vi "Hard Link To Source.vi"(8 "Error In":errorcluster, 11 "Configuration in":T1) -> (0 "Error Out":errorcluster, 2 "Files Added To Source":path[](array[path]), 3 "Configuration out":T1)   [LabVIEW 2011, in "LVH-Build-Tools.lvlib"]
doc: "Scan through all components and create hardlinks in source for any files that exist in install but not source."
uses:
  <vilib>/LabVIEW Hacker/Build Tools/LVH-Build-Tools.lvlib
  Type Defs/Configuration.ctl
  Type Defs/Install Configuration.ctl
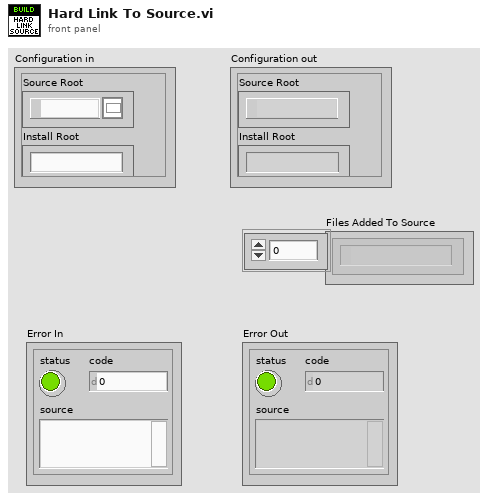
[diagram p1: front panel]
types:
  T1 = typedef "LVH-Build-Tools.lvlib/Configuration.ctl" = cluster{"Source Root":path, "Install Root":string, "Components":string[], "Ignore":string[], "Config Files":path[], "LV Directories":path[], "Install Paths":T2}
  T2 = typedef "LVH-Build-Tools.lvlib/Install Configuration.ctl" = cluster{"LabVIEW Directory":path, "Project Source Config":path}
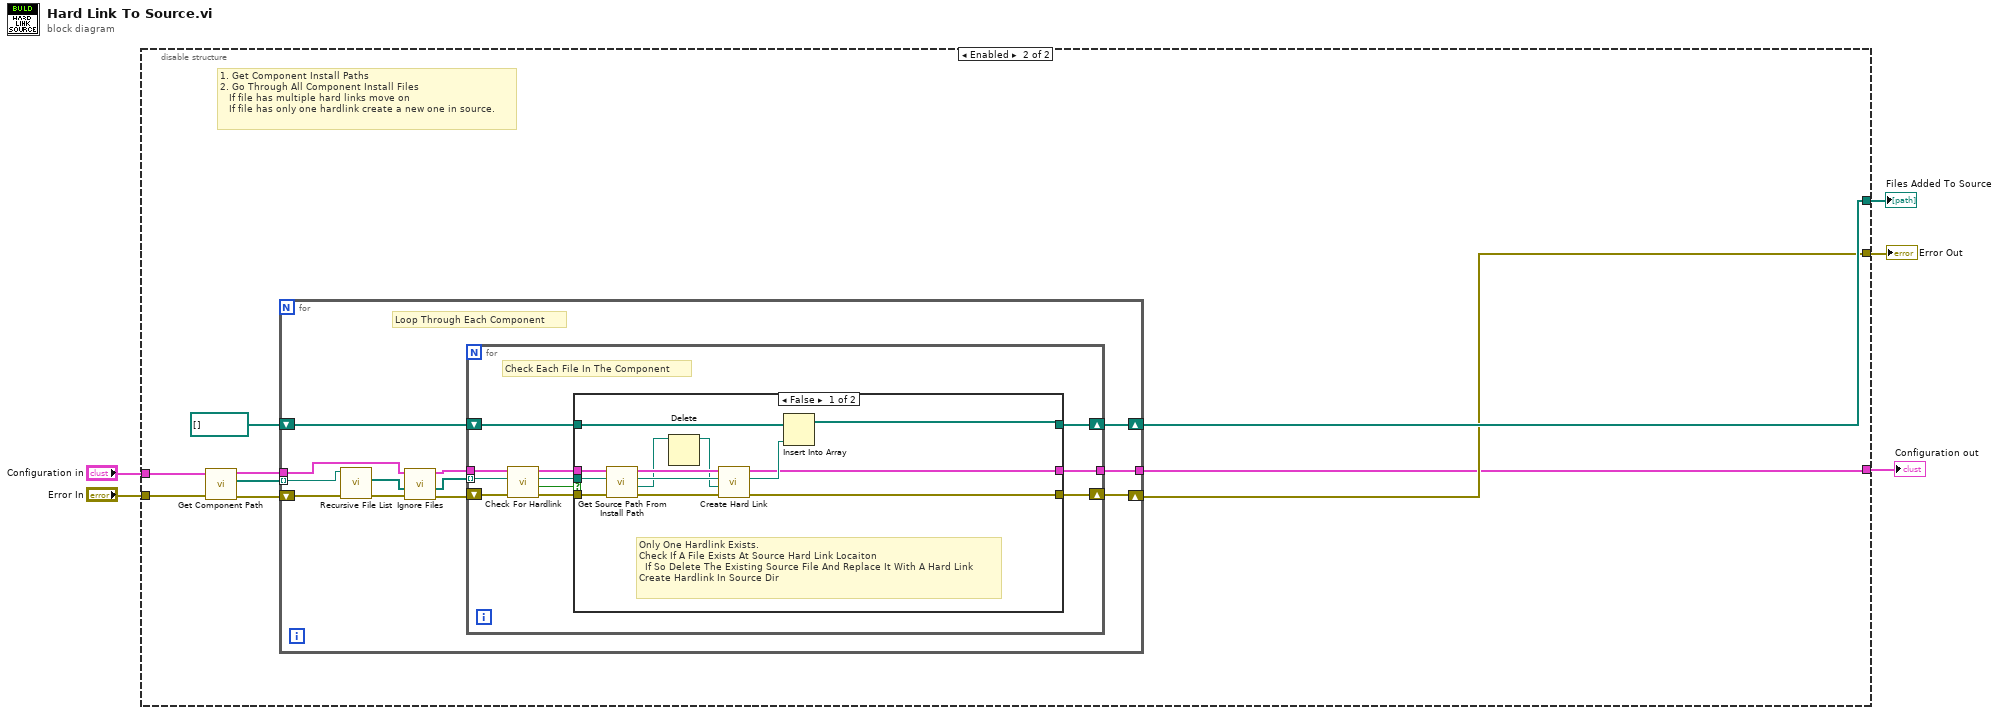
[diagram p0: block diagram]
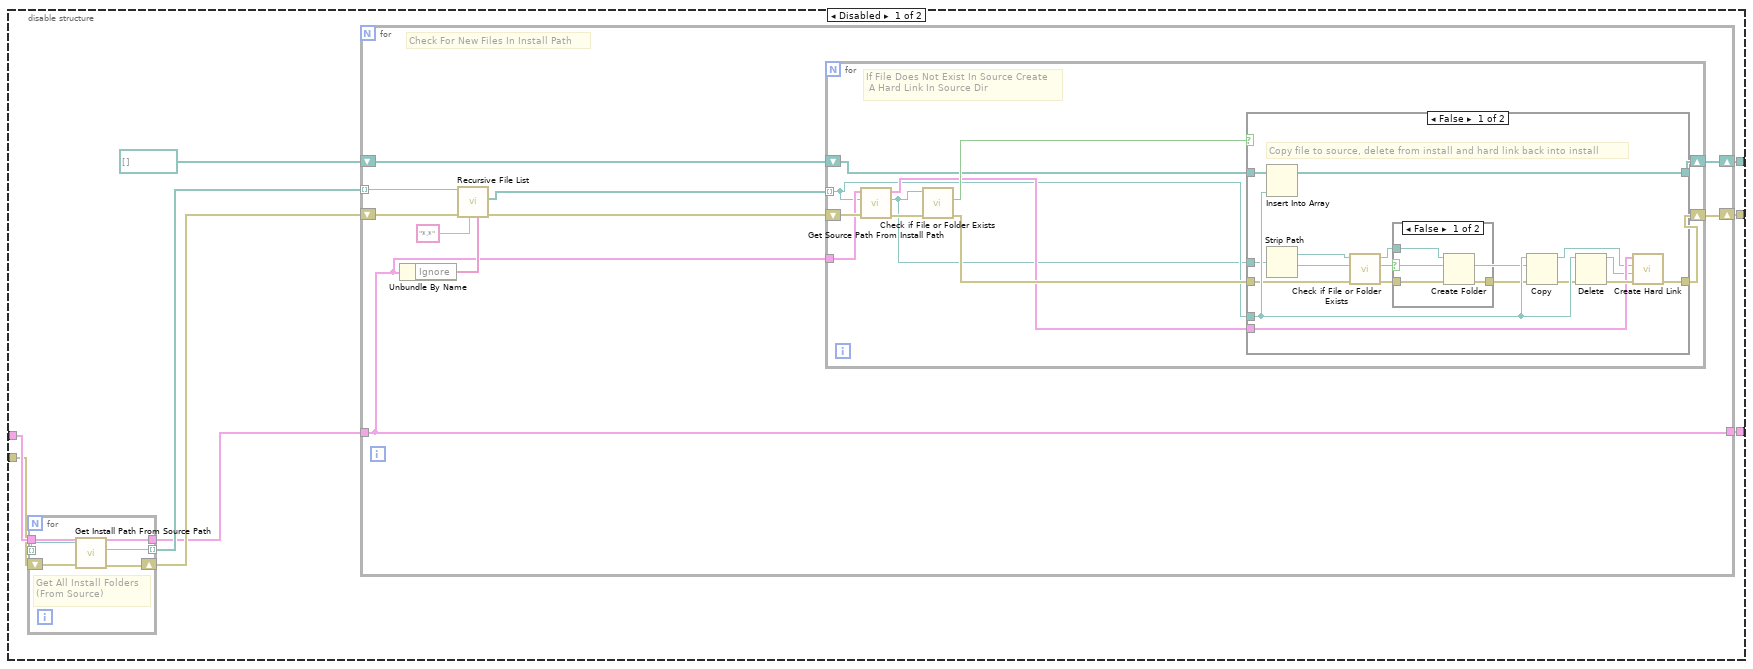
[diagram p2: hidden frame]
diagram:
  n1 = disable-structure shown="Enabled" {
    disable-tunnel: "Configuration in" -> [w11 w73]
    disable-tunnel: "Error In" -> [w10 w72]
    disable-tunnel: [w9 w65] -> w3
    disable-tunnel: [w8 w66] -> w2
    disable-tunnel: [w7 w67] -> w1
    frame Disabled {
      n2 = for {
        tunnel: w11 -> [w20]
        tunnel: [w19] -> w12
        tunnel: [w17] -> w14 mode=indexing
        shift-right: [w18] -> w13
        shift-left: w10 -> [w21]
        tunnel: [w16] -> w15 mode=indexing
        # "Get All Install Folders \n(From Source)"
        n3 = call "Get Install Path From Source Path.vi"("Error In"=w21, "Source File Path"=w17, "Configuration"=w20) -> ("Error Out"=w18:errorcluster, "Install File Path"=w16:path, "Configuration"=w19:T1)  [unwired: 5 in, 1 out]
      }
      n4 = for {
        tunnel: w15 -> [w31] mode=indexing
        shift-right: [w25] -> w8
        shift-left: w13 -> [w30]
        tunnel: w12 -> [w22]
        tunnel: [w22] -> w9
        shift-right: [w23] -> w7
        shift-left: path[] [] -> [w24]
        # "Check For New Files In Install Path"
        n5 = Unbundle By Name(w22) -> ("Ignore"=w28:string[])
        n6 = call <vilib>:"Recursive File List.vi"("Folders to Exclude"=w28, "pattern"="*.*", "error in (no error)"=w30, "Folder Path"=w31) -> ("error out"=w27:errorcluster, "All Files in Dir"=w26:path[])  [unwired: 3 in, 3 out]
        n7 = for {
          tunnel: w26 -> [w33] mode=indexing
          shift-right: [w38] -> w25
          shift-left: w27 -> [w42]
          shift-right: [w36] -> w23
          shift-left: w24 -> [w37]
          tunnel: w22 -> [w35]
          # "If File Does Not Exist In Source Create\n A Hard Link In Source Dir"
          n8 = call "Get Source Path From Install Path.vi"("Error In"=w42, "Install File Path"=w33, "Configuration"=w35) -> ("Error Out"=w41:errorcluster, "Install File Path"=w32:path, "Configuraiton"=w34:T1)  [unwired: 5 in, 1 out]
          n9 = call <vilib>:"Check if File or Folder Exists.vi"("error in (no error)"=w41, "path"=w32) -> ("error out"=w39:errorcluster, "file or folder exists?"=w40:bool)  [unwired: 7 in, 1 out]
          n10 = case shown="False" w40 {
            tunnel: w33 -> [w57 _]
            tunnel: w39 -> [w48 w64]
            tunnel: [w51 w64] -> w38
            tunnel: w37 -> [w58 w63]
            tunnel: [w50 w63] -> w36
            tunnel: w34 -> [w54 _]
            tunnel: w32 -> [w43 _]
            frame False {
              # "Copy file to source, delete from install and hard link back into install"
              n11 = Insert Into Array(array=w58, new element=w57) -> (w50:path[])  [unwired: 1 in]
              n12 = Strip Path(path=w43) -> (stripped path=w49:path)  [unwired: 1 out]
              n13 = call <vilib>:"Check if File or Folder Exists.vi"("error in (no error)"=w48, "path"=w49) -> ("error out"=w45:errorcluster, "file or folder exists?"=w47:bool, "dup path"=w46:path)  [unwired: 7 in]
              n14 = case shown="False" w47 {
                tunnel: w46 -> [w61 _]
                tunnel: w45 -> [w60 w62]
                tunnel: [w59 w62] -> w44
                frame False {
                  n15 = Create Folder(path (use dialog)=w61, error in=w60) -> (error out=w59:errorcluster)  [unwired: 1 in, 2 out]
                }
                frame True {
                }
              }
              n16 = Copy(8:w44, 10:w43, 11:w57) -> (0:w56:errorcluster, 3:w53:path)  [unwired: 2 in, 1 out]
              n17 = Delete(path (use dialog)=w57, error in=w56) -> (deleted path=w52:path, error out=w55:errorcluster)  [unwired: 3 in, 1 out]
              n18 = call "Create Hard Link.vi"("Error In"=w55, "Link Destination Path"=w52, "Existing File Path"=w53, "Configuration"=w54) -> ("Error Out"=w51:errorcluster)  [unwired: 5 in, 2 out]
            }
            frame True {
              # "File Already Exists In Source\nNo Need To Create Hard Link"
            }
          }
        }
      }
    }
    frame Enabled {
      # "1. Get Component Install Paths\n2. Go Through All Component Install Files\n   If file has multiple hard links move on\n   If file has only one hardlink create a new one in source."
      n19 = call "Get Component Path.vi"("Error In"=w72, "Configuration"=w73) -> ("Error Out"=w70:errorcluster, "Component Install Paths"=w69:path[], "Configuration"=w71:T1)  [unwired: 7 in]
      n20 = for {
        tunnel: w71 -> [w77]
        tunnel: w69 -> [w85] mode=indexing
        shift-right: [w82] -> w67
        shift-left: path[] [] ("array") -> [w83]
        shift-right: [w81] -> w66
        shift-left: w70 -> [w84]
        tunnel: [w80] -> w65
        # "Loop Through Each Component"
        n21 = call <vilib>:"Recursive File List.vi"("error in (no error)"=w84, "Folder Path"=w85) -> ("error out"=w79:errorcluster, "All Files in Dir"=w74:path[])  [unwired: 5 in, 3 out]
        n22 = call "Ignore Files.vi"("Error In"=w79, "All Files"=w74, "Configuration"=w77) -> ("Error Out"=w78:errorcluster, "All Files"=w75:path[], "Configuration"=w76:T1)  [unwired: 5 in, 1 out]
        n23 = for {
          tunnel: w76 -> [w95]
          shift-right: [w89] -> w82
          shift-left: w83 -> [w90]
          shift-right: [w88] -> w81
          shift-left: w78 -> [w96]
          tunnel: [w87] -> w80
          tunnel: w75 -> [w86] mode=indexing
          # "Check Each File In The Component"
          n24 = call "Check For Hardlink.vi"("Error In"=w96, "File Path"=w86, "Configuration"=w95) -> ("Error Out"=w91:errorcluster, "Multiple Hardlinks"=w94:bool, "Dup File Path"=w93:path, "Configuration"=w92:T1)  [unwired: 5 in]
          n25 = case shown="False" w94 {
            tunnel: w93 -> [w106 _]
            tunnel: w92 -> [w109 w111]
            tunnel: w91 -> [w108 w112]
            tunnel: w90 -> [w103 w110]
            tunnel: [w102 w110] -> w89
            tunnel: [w101 w112] -> w88
            tunnel: [w100 w111] -> w87
            frame False {
              # "Only One Hardlink Exists.\nCheck If A File Exists At Source Hard Link Locaiton\n  If So Delete The Existing Source File And Replace It With A Hard Link\nCreate Hardlink In Source Dir"
              n26 = call "Get Source Path From Install Path.vi"("Error In"=w108, "Install File Path"=w106, "Configuration"=w109) -> ("Error Out"=w97:errorcluster, "Source File Path"=w99:path, "Install File Path"=w105:path, "Configuraiton"=w107:T1)  [unwired: 5 in]
              n27 = Delete(path (use dialog)=w99) -> (deleted path=w98:path)  [unwired: 4 in, 2 out]
              n28 = call "Create Hard Link.vi"("Error In"=w97, "Link Destination Path"=w98, "Existing File Path"=w105, "Configuration"=w107) -> ("Error Out"=w101:errorcluster, "Created Hardlink Path"=w104:path, "Configuration"=w100:T1)  [unwired: 5 in]
              n29 = Insert Into Array(array=w103, new element=w104) -> (w102:path[])  [unwired: 1 in]
            }
            frame True {
              # "Multiple Hardlinks Exits\nNothing To Do"
            }
          }
        }
      }
    }
  }
  "Configuration out" <- w3
  "Error Out" <- w2
  "Files Added To Source" <- w1
